vi "analog_to_radian.vi"(1 "Offset":dbl, 2 "Analog signal":dbl) -> (0 "Radians":dbl)   [LabVIEW 2021]
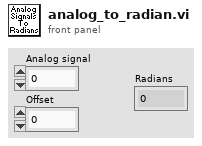
[diagram p1: front panel]
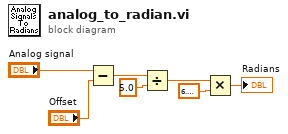
[diagram p0: block diagram]
diagram:
  n1 = Subtract(x="Analog signal", y="Offset") -> (x-y=w7:dbl)
  n2 = Divide(x=w7, y=5.0) -> (x/y=w5:dbl)
  n3 = Multiply(x=w5, y=6.283185307179586) -> (x*y=→"Radians":dbl)
